vi "reverse.u64.vi"(11 "U64.in":u64=18374686479671623680 format="%.0x") -> (3 "U64.reversed":u64=255 format="%.0x")   [LabVIEW 2020, in "fpganow.common.fpga.lvlib"]
uses:
  fpganow.common.fpga.lvlib
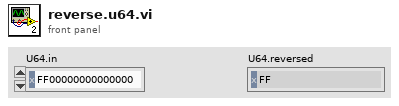
[diagram p1: front panel]
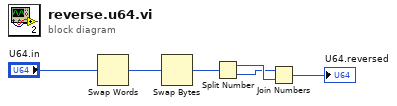
[diagram p0: block diagram]
diagram:
  n1 = Swap Words(1:"U64.in") -> (0:w5:u64)
  n2 = Swap Bytes(anything=w5) -> (byte swapped=w4:u64)
  n3 = Split Number(x=w4) -> (hi(x)=w3:u32, lo(x)=w2:u32)
  n4 = Join Numbers(hi=w2, lo=w3) -> ((hi.lo)=→"U64.reversed":u64)
